vi "set pockels cell.vi"(8 "error in (no error)":errorcluster, 11 "ImagingModeSPIM in":refnum<class "ImagingModeSPIM.lvclass">) -> (0 "error out":errorcluster, 3 "ImagingModeSPIM out":refnum<class "ImagingModeSPIM.lvclass">)   [LabVIEW 2012, in "ImagingModeSPIM.lvclass"]
uses:
  ImagingModeSPIM.lvclass
  ImagingModeSPIM.lvclass/ImagingModeSPIM.ctl
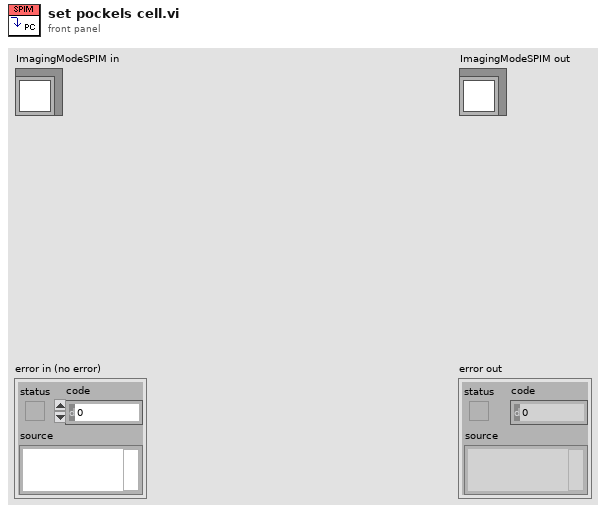
[diagram p1: front panel]
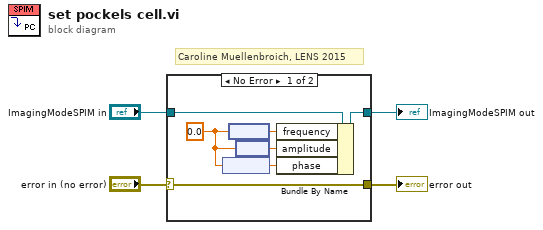
[diagram p0: block diagram]
diagram:
  # "Caroline Muellenbroich, LENS 2015"
  n1 = case shown="No Error" "error in (no error)" {
    selector: "error in (no error)" -> [w11 w13]
    tunnel: [w11 w13] -> w3
    tunnel: [w9 w12] -> w1
    tunnel: "ImagingModeSPIM in" -> [w10 w12]
    frame No Error {
      w8 = 0.0 ("settings.Pockels Cell.frequency")
      n2 = node(w8) -> (w7:dbl[unit])
      n3 = node(w8) -> (w5:dbl[unit])
      n4 = node(w8) -> (w6:dbl[unit])
      n5 = Bundle By Name(cluster=w10, "frequency"=w5, "amplitude"=w6, "phase"=w7) -> (w9:refnum<class "ImagingModeSPIM.lvclass">)
    }
    frame Error {
    }
  }
  "error out" <- w3
  "ImagingModeSPIM out" <- w1
